vi "MeasureIV.vi"(5 "Junction Name":string, 6 "UiDefinition":T1, 7 ".NET Refnum":refnum<k24>, 8 "new file path (Not A Path if cancelled)":path, 9 "appended path":path, 11 ".NET Refnum in":refnum<k24>) -> (0 "error out":errorcluster)   [LabVIEW 2020]
uses:
  D:/LabviewDXFViewer/LabviewDXFViewer/bin/Release/LabviewDXFViewer.exe
  LabviewDXFViewer/bin/Release/LabviewDXFViewer.exe
  UIReferences.ctl
  <vilib>/Utility/file.llb/Write Delimited Spreadsheet (string).vi
  <vilib>/Utility/file.llb/Write Delimited Spreadsheet (DBL).vi
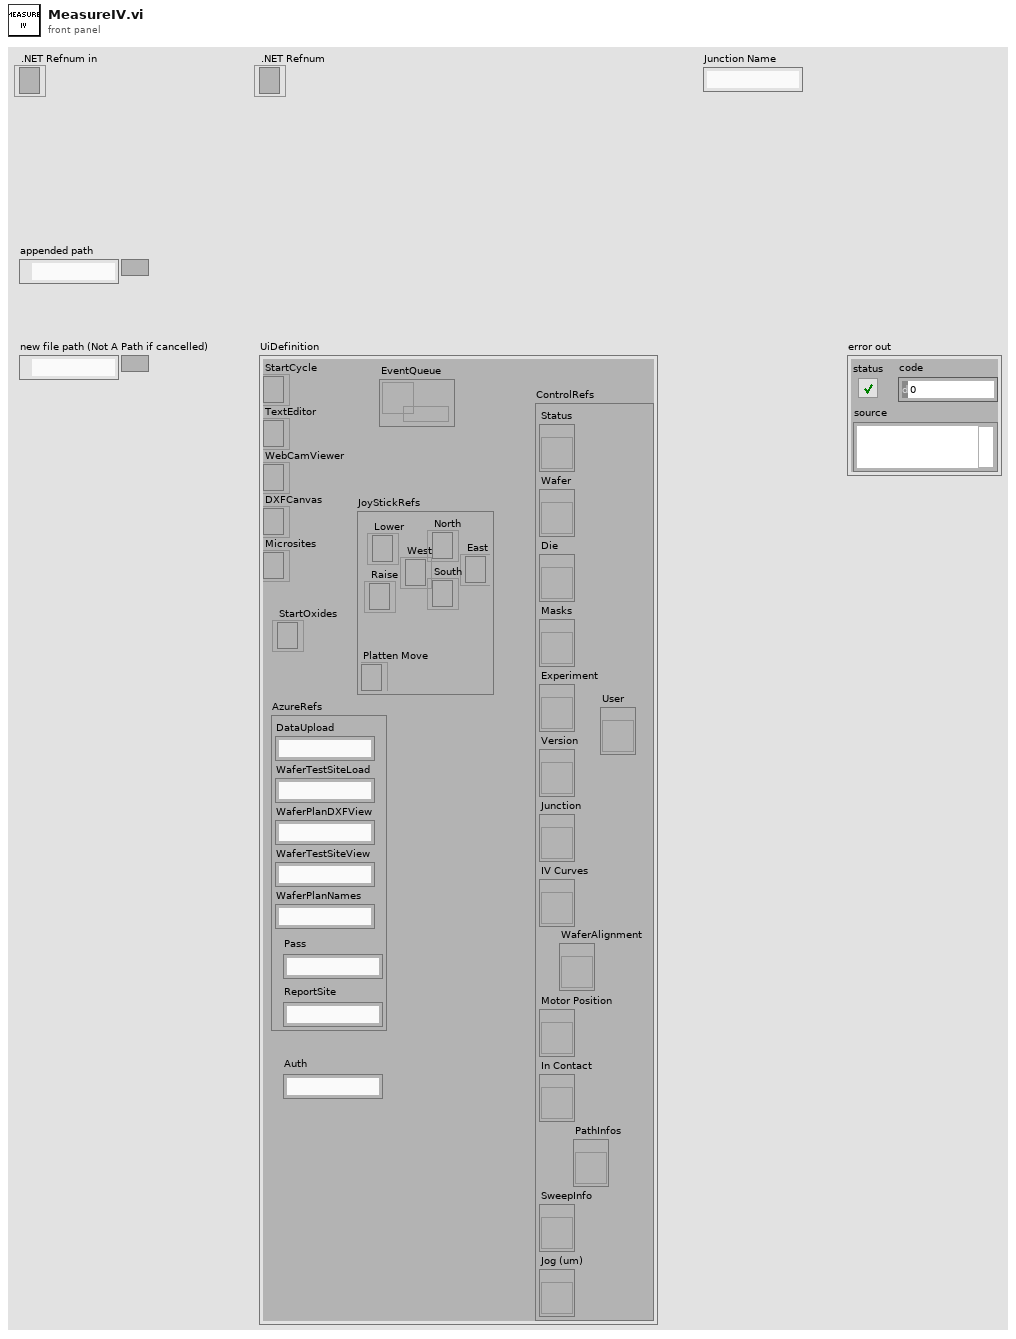
[diagram p1: front panel]
types:
  T1 = typedef "UIReferences.ctl" = cluster{"StartCycle":refnum<k24>, "TextEditor":refnum<k24>, "WebCamViewer":refnum<k24>, "DXFCanvas":refnum<k24>, "Microsites":refnum<k24>, "JoyStickRefs":cluster{"North":refnum<k24>, "Lower":refnum<k24>, "Raise":refnum<k24>, "Platten Move":refnum<k24>, "West":refnum<k24>, "East":refnum<k24>, "South":refnum<k24>}, "AzureRefs":cluster{"DataUpload":string, "WaferTestSiteLoad":string, "WaferPlanDXFView":string, "WaferTestSiteView":string, "WaferPlanNames":string, "Pass":string, "ReportSite":string}, "ControlRefs":cluster{"Status":refnum<vi>, "Wafer":refnum<vi>, "Die":refnum<vi>, "Masks":refnum<vi>, "Experiment":refnum<vi>, "Version":refnum<vi>, "Junction":refnum<vi>, "IV Curves":refnum<vi>, "Motor Position":refnum<vi>, "In Contact":refnum<vi>, "SweepInfo":refnum<vi>, "Jog (um)":refnum<vi>, "PathInfos":refnum<vi>, "User":refnum<vi>, "WaferAlignment":refnum<vi>}, "EventQueue":refnum<queue>, "StartOxides":refnum<k24>, "Auth":string}
  T2 = typedef "CapacitanceInfos.ctl" = cluster{"Conductance":dbl, "CapacitanceIV":dbl, "Intercept":dbl, "CapacitanceSW":dbl, "Sum":dbl, "CapacitanceInfos":T3[], "CapacitancePhase":dbl, "dC/dV":dbl, "Function":string, "OtherInfo":dbl[][]}
  T3 = typedef "CapacitanceRecord.ctl" = cluster{"Freq":dbl, "Vpp":dbl, "PhaseS":dbl, "Irms":dbl, "PhaseC":dbl, "Theta":dbl, "VDrive":dbl, "Capacitance":dbl, "Other":dbl}
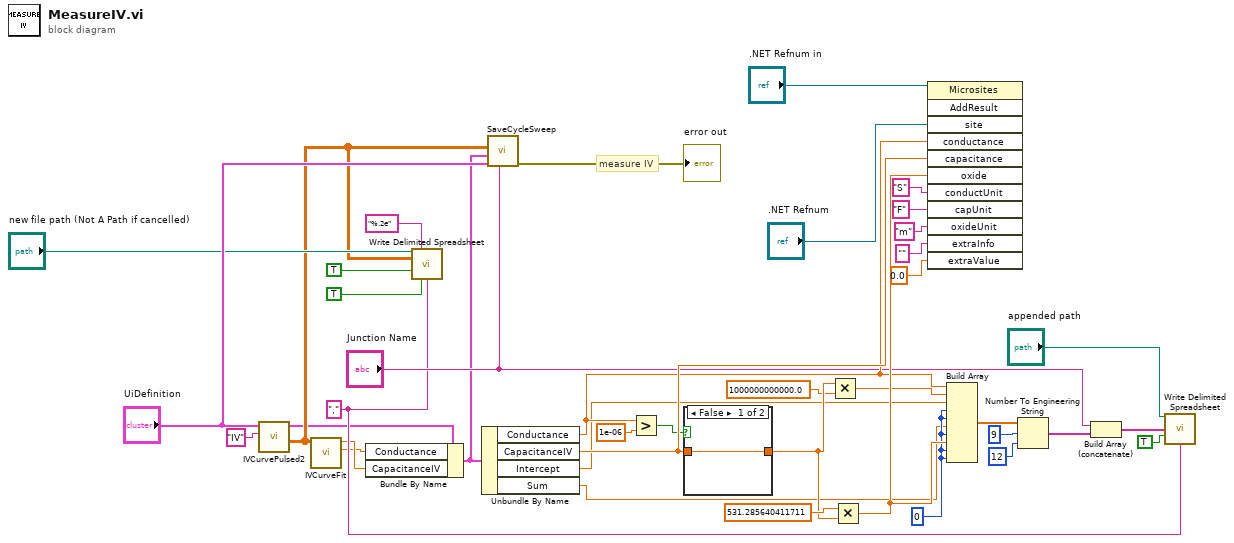
[diagram p0: block diagram]
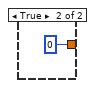
[diagram p2: hidden frame]
diagram:
  w9 = "," ("delimiter (\\t)")
  w35 = 0
  # "measure IV"
  n1 = call "IVCurvePulsed2.vi"("Program"="IV", "UiDefinition"="UiDefinition") -> ("appended array"=w5:dbl[][], "InfoCluster"=w4:T2)  [unwired: 8 in]
  n2 = call "IVCurveFit.vi"("IVData"=w5) -> ("Conductance"=w1:dbl, "Capacitance"=w2:dbl)  [unwired: 8 in, 1 out]
  n3 = Bundle By Name(cluster=w4, "Conductance"=w1, "CapacitanceIV"=w2) -> (w3:T2)
  n4 = call-poly <vilib>:"Write Delimited Spreadsheet.vi"("file path (dialog if empty)"="new file path (Not A Path if cancelled)", "format (%.3f)"="%.2e", "2D data"=w5, "append to file? (new file:F)"=TRUE, "transpose? (no:F)"=TRUE, "delimiter (\\t)"=w9) -> ()  [unwired: 8 in, 2 out]
  n5 = Unbundle By Name(w3) -> ("Conductance"=w36:dbl, "CapacitanceIV"=w37:dbl, "Intercept"=w19:dbl, "Sum"=w20:dbl)
  n6 = call "SaveCycleSweep.vi"("JunctionName"="Junction Name", "UiDefinition 2"="UiDefinition", "InfoCluster"=w3, "appended array"=w5) -> ("error out"=→"error out":errorcluster)  [unwired: 7 in]
  n7 = Greater?(x=w36, y=1e-06) -> (0:w23:bool)
  n8 = case shown="False" w23 {
    tunnel: [w41 0] -> w38
    tunnel: w37 -> [w41 _]
    frame False {
    }
    frame True {
    }
  }
  n9 = Multiply(x=w38, y=1000000000000.0) -> (x*y=w21:dbl)
  n10 = Multiply(x=531.285640411711, y=w38) -> (x*y=w40:dbl)
  n11 = invoke class="Microsites" method="AddResult"(reference=".NET Refnum in", "site"=".NET Refnum", "conductance"=w36, "capacitance"=w37, "oxide"=w40, "conductUnit"="S", "capUnit"="F", "oxideUnit"="m" ("interceptUnit"), "extraInfo"="", "extraValue"=0.0) -> ()  [unwired: 2 in, 12 out]
  n12 = Build Array(w36, w21, w19, w35, w35, w20, w35, w40, w35, w35) -> (w18:dbl[])
  n13 = Number To Engineering String(2:i16 12 ("precision (6)"), 3:i16 9 ("width (-)"), 4:w18) -> (0:w11:string[])  [unwired: 1 in]
  n14 = Build Array (concatenate)("Junction Name", w11) -> (w13:string[])
  n15 = call-poly <vilib>:"Write Delimited Spreadsheet.vi"("file path (dialog if empty)"="appended path", "1D data"=w13, "append to file? (new file:F)"=TRUE, "delimiter (\\t)"=w9) -> ()  [unwired: 10 in, 2 out]
